vi "one_button.vi"(7 "callee":refnum<vi>, 8 "error in (no error)":errorcluster, 11 "configuration 2":T1) -> (0 "error out":errorcluster, 3 "dialog_selection":T2)   [LabVIEW 2015, in "lv-dialog-interfaces.lvlib"]
uses:
  lv-dialog-interfaces.lvlib
  private/_controls/hmi_references.ctl
  private/_controls/dialog_type.ctl
  <vilib>/event_ctls.llb/eventvkey.ctl
  private/_controls/configuration.ctl
  lv-dialog/api/v1/public/_controls/dialog_selection.ctl
  lv-dialog/api/v1/v1.lvlib
panel:
  out "dialog":string
  in  "button_1":bool
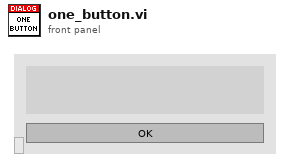
[diagram p1: front panel]
types:
  T1 = cluster{"dialog_text":string, "boolean_text_1":string}
  T2 = typedef "lv-dialog.lvlib/v1.lvlib/dialog_selection.ctl" = enum16{"null", "panel_closed", "button_1", "button_2", "button_3", "cancelled"}
  T3 = typedef "lv-dialog-interfaces.lvlib/dialog_type.ctl" = enum16{"null", "one_button", "two_button", "three_button", "confirmation", "busy_wait", "error", "busy_wait_embed", "combo_box", "data_entry_string", "data_entry_numeric"}
  T4 = typedef "lv-dialog-interfaces.lvlib/configuration.ctl" = cluster{"dialog_text":string, "boolean_text_1":string, "boolean_text_2":string, "boolean_text_3":string, "inner_color":u32, "outer_color":u32, "wait_s":dbl, "error_status":bool, "error_source":string, "error_details":string, "string []":string[], "custom_entry":bool}
  T5 = typedef "lv-dialog-interfaces.lvlib/hmi_references.ctl" = cluster{"vi_reference":refnum<vi>, "caller":refnum<vi>, "dialog":refnum<vi>, "button_1":refnum<vi>, "button_2":refnum<vi>, "button_3":refnum<vi>, "busy":refnum<vi>, "error_glyph":refnum<vi>, "error_source":refnum<vi>, "error_text":refnum<vi>, "combo_box":refnum<vi>}
  T6 = typedef "eventvkey.ctl" = enum16{"ASCII", "Enter", "Return", "Shift", "Ctrl", "Alt", "Cmd", "Opt", "Caps", "NumLock", "Clear", "Break", "Up", "Down", "Left", "Right", "Insert", "Delete", "Home", "End", "PageUp", "PageDown", "Escape", "Help", "Pause", "ScrollLock", "F1", "F2", "F3", "F4", "F5", "F6", "F7", "F8", "F9", "F10", "F11", "F12", "F13", "F14", "F15", "F16", "F17", "F18", "F19", "F20", "F21", "F22", "F23", "F24", "Play", "VolumeUp", "VolumeDown", "Mute", "Two Byte Char"}
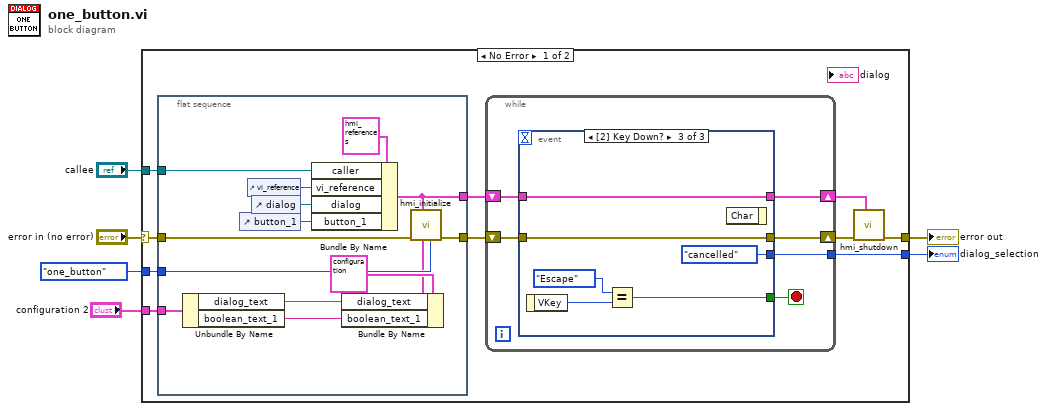
[diagram p0: block diagram]
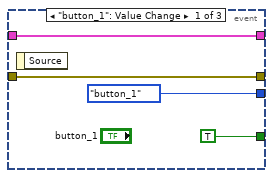
[diagram p2: hidden frame]
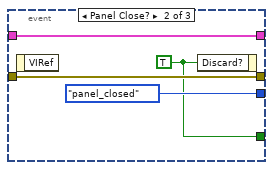
[diagram p3: hidden frame]
diagram:
  n1 = case shown="No Error" "error in (no error)" {
    selector: "error in (no error)" -> [w16 w51]
    tunnel: dialog_type."one_button" ("dialog_type") -> [w15 _]
    tunnel: [w13 _] -> w4
    tunnel: "callee" -> [w12 _]
    tunnel: [w10 w51] -> w2
    tunnel: "configuration 2" -> [w7 _]
    frame No Error {
      n2 = flat-sequence {
        tunnel: w16 -> [w24]
        tunnel: w15 -> [w26]
        tunnel: [w25] -> w14
        tunnel: w12 -> [w23]
        tunnel: [w22] -> w9
        tunnel: w7 -> [w21]
        frame #0 {
          n3 = Unbundle By Name(w21) -> ("dialog_text"=w18:string, "boolean_text_1"=w17:string)
          n4 = control-ref of="button_1"() -> (w28:refnum<vi>)
          n5 = control-ref of="vi_reference"() -> (w30:refnum<vi>)
          n6 = control-ref of="dialog"() -> (w29:refnum<vi>)
          n7 = Bundle By Name(cluster=T5 {"vi_reference"=refnum, "caller"=refnum, "dialog"=refnum, "button_1"=refnum, "button_2"=refnum, "button_3"=refnum, "busy"=refnum, "error_glyph"=refnum, "error_source"=refnum, "error_text"=refnum, "combo_box"=refnum}, "caller"=w23, "vi_reference"=w30, "dialog"=w29, "button_1"=w28) -> (w22:T5)
          n8 = Bundle By Name(cluster=T4 {"dialog_text"="", "boolean_text_1"="", "boolean_text_2"="", "boolean_text_3"="", "inner_color"=16711680, "outer_color"=6618880, "wait_s"=nan, "error_status"=FALSE, "error_source"="", "error_details"="", "string []"=[], "custom_entry"=FALSE} ("configuration"), "dialog_text"=w18, "boolean_text_1"=w17) -> (w19:T4)
          n9 = call "hmi_initialize.vi"("dialog_type"=w26, "configuration"=w19, "references"=w22, "error in (no error)"=w24) -> ("error out"=w25:errorcluster)  [unwired: 7 in]
        }
      }
      n10 = while {
        tunnel: [w34] -> w13
        shift-right: [w35] -> w11
        shift-left: w14 -> [w36]
        shift-right: [w32] -> w8
        shift-left: w9 -> [w33]
        stop <- w31 stop-if-true
        n11 = event shown="[2] Key Down?" {
          selector: _ -> [_ _ _]
          dyn-events: _ -> [_ _ _]
          timeout: _ -> [_ _ _]
          tunnel: w36 -> [w40 w44 w45]
          tunnel: [w40 w44 w45] -> w35
          tunnel: [dialog_selection."button_1" ("dialog_selection") dialog_selection."panel_closed" ("dialog_selection") dialog_selection."cancelled" ("dialog_selection")] -> w34
          tunnel: w33 -> [w38 w42 w50]
          tunnel: [w38 w42 w50] -> w32
          tunnel: [TRUE w41 w47] -> w31
          event "button_1": Value Change {
            n12 = event-data() -> ()  [unwired: 1 in, 1 out]
          }
          event Panel Close? {
            w41 = TRUE ("Discard?")
            n13 = event-data() -> ()  [unwired: 1 in, 1 out]
            n14 = event-data("Discard?"=w41) -> ()  [unwired: 1 in, 1 out]
          }
          event Key Down? {
            n15 = event-data() -> ("VKey"=w49:T6)  [unwired: 1 in]
            n16 = Equal?(x=eventvkey."Escape" ("VKey"), y=w49) -> (x = y?=w47:bool)
            n17 = event-data() -> ()  [unwired: 2 in, 1 out]
          }
        }
      }
      n18 = call "hmi_shutdown.vi"("references"=w8, "error in (no error)"=w11) -> ("error out"=w10:errorcluster)  [unwired: 9 in]
    }
    frame Error {
    }
  }
  "error out" <- w2
  "dialog_selection" <- w4
